vi "SINAD Analyzer.vi"   [LabVIEW 2020, in "NI_MAPro.lvlib"]
doc: "Takes a signal in and performs a full Signal in Noise and Distortion (SINAD) analysis, including measuring the fundamental frequency tone and returning the fundamental frequency and SINAD level in dB. Wire data to the <B>signal in</B> input to determine the polymorphic instance to use or manually select the instance."
uses:
  NI_MAPro.lvlib
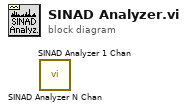
[diagram p0: block diagram]
diagram:
  n1 = call "SINAD Analyzer N Chan.vi"() -> ()  [unwired: 6 in, 6 out]
  n2 = call "SINAD Analyzer 1 Chan.vi"() -> ()  [unwired: 6 in, 6 out]
